vi "Write Single Coil.vi"(8 "error in (no error)":errorcluster, 9 "coil value":bool, 10 "address":u16, 11 "Modbus master in":refnum<class "Modbus Master.lvclass">) -> (0 "error out":errorcluster, 3 "Modbus master out":refnum<class "Modbus Master.lvclass">)   [LabVIEW 2021, in "Modbus Master.lvclass"]
doc: "Writes a value to a single coil."
uses:
  Modbus Master.lvclass
  D:/my_projects/projects/Algorithms/Labview/21/Modbus_v121c/API/Modbus API.lvclass
  Modbus API.lvclass/Modbus API.ctl
  Network Protocol/Network Protocol.lvclass/Network Protocol.ctl
  Modbus Master.lvclass/Modbus Master.ctl
  Transmission Data Unit/Transmission Data Unit.lvclass
  Master Function Definition/Master Function Definition.lvclass
  Modbus API.lvclass
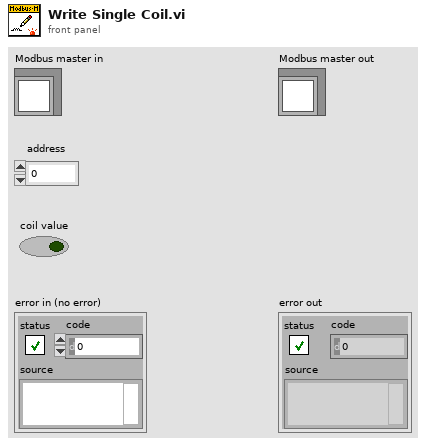
[diagram p1: front panel]
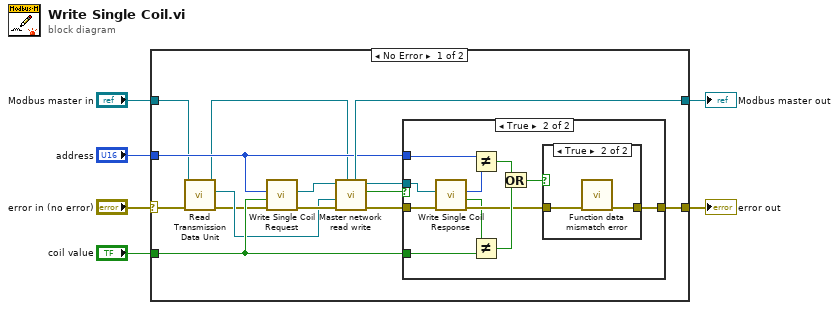
[diagram p0: block diagram]
diagram:
  n1 = case shown="No Error" "error in (no error)" {
    selector: "error in (no error)" -> [w9 w37]
    tunnel: "Modbus master in" -> [w10 w36]
    tunnel: [w19 w37] -> w3
    tunnel: [w14 w36] -> w2
    tunnel: "address" -> [w12 _]
    tunnel: "coil value" -> [w18 _]
    frame No Error {
      n2 = call "Read Transmission Data Unit.vi"("error in"=w9, "Modbus instance in"=w10) -> ("error out"=w7:errorcluster, "transmission data unit"=w13:refnum<class "Transmission Data Unit.lvclass">, "Modbus instance out"=w8:refnum<class "Modbus Master.lvclass">)  [unwired: 7 in]
      n3 = call "Write Single Coil Request.vi"("error in"=w7, "Coil Value"=w18, "Starting Address"=w12) -> ("error out"=w20:errorcluster, "modbus data unit out"=w16:refnum<class "Modbus Data Unit.lvclass">)  [unwired: 7 in]
      n4 = call "Master network read write.vi"("Modbus master in"=w8, "error in (no error)"=w20, "transmission data unit in"=w13, "Modbus data unit in"=w16) -> ("error out"=w17:errorcluster, "PDU valid?"=w11:bool, "Modbus data unit out"=w15:refnum<class "Modbus Data Unit.lvclass">, "Modbus master out"=w14:refnum<class "Modbus Master.lvclass">)  [unwired: 4 in]
      n5 = case shown="True" w11 {
        tunnel: [w21 w31] -> w19
        tunnel: w18 -> [_ w23]
        tunnel: w17 -> [w21 w27]
        tunnel: w15 -> [_ w26]
        tunnel: w12 -> [_ w24]
        frame False {
        }
        frame True {
          n6 = call "Write Single Coil Response.vi"("error in"=w27, "modbus data unit in"=w26) -> ("error out"=w25:errorcluster, "Coil Value"=w22:bool, "Address"=w28:u16)  [unwired: 7 in]
          n7 = Not Equal?(x=w24, y=w28) -> (x != y?=w30:bool)
          n8 = Not Equal?(x=w22, y=w23) -> (x != y?=w29:bool)
          n9 = Or(x=w30, y=w29) -> (x .or. y?=w32:bool)
          n10 = case shown="True" w32 {
            tunnel: [w33 w35] -> w31
            tunnel: w25 -> [w33 w34]
            frame False {
            }
            frame True {
              n11 = call "Function data mismatch error.vi"("error in (no error)"=w34) -> ("error out"=w35:errorcluster)  [unwired: 10 in]
            }
          }
        }
      }
    }
    frame Error {
    }
  }
  "error out" <- w3
  "Modbus master out" <- w2
